vi "Delete Float32 DVR.vi"(8 "error in (no error)":errorcluster, 11 "Float32 DVR in":refnum<data-value>) -> (0 "error out":errorcluster, 3 "Float32 out":refnum<class "Float32.lvclass">)   [LabVIEW 2015, in "MDSplus.lvlib" / "Float32.lvclass"]
uses:
  <vilib>/MDSplus/Classes/Data_Class/Scalar_Class/Float32_Class/Float32.lvclass
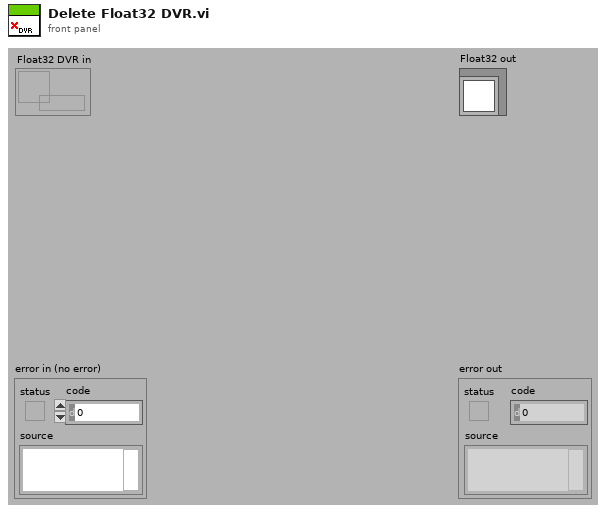
[diagram p1: front panel]
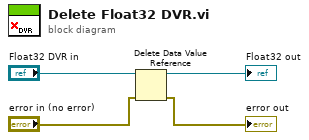
[diagram p0: block diagram]
diagram:
  n1 = Delete Data Value Reference(data value reference="Float32 DVR in", error in="error in (no error)") -> (data value=→"Float32 out":refnum<class "Float32.lvclass">, error out=→"error out":errorcluster)
